vi "Read I2C.vi"(5 "Address":u8, 6 "NoStop (F)":bool, 7 "Bus":u8, 8 "error in (no error)":errorcluster, 9 "Len":u8, 11 "VISA resource name in":refnum<visa-resource-name>) -> (0 "error out":errorcluster, 1 "Data":string, 3 "VISA resource name":refnum<visa-resource-name>)   [LabVIEW 2024, in "CTIPicoVISA.lvlib"]
uses:
  CTIPicoVISA.lvlib
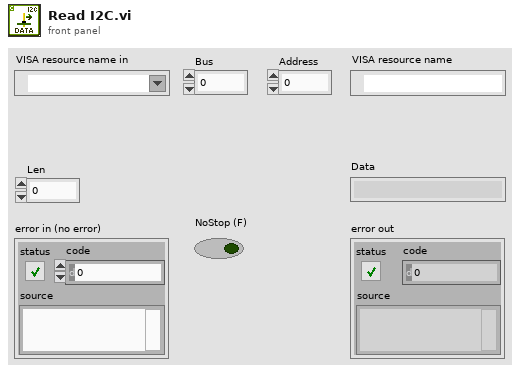
[diagram p1: front panel]
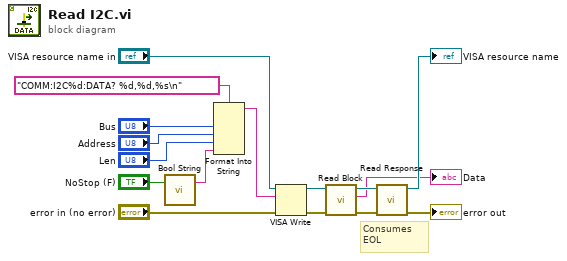
[diagram p0: block diagram]
diagram:
  # "Consumes EOL"
  n1 = call "Bool String.vi"("Bool"="NoStop (F)") -> ("String"=w3:string)  [unwired: 6 in]
  n2 = Format Into String(format string="COMM:I2C%d:DATA? %d,%d,%s\n", "Bus", "Address", "Len", w3) -> (resulting string=w1:string)  [unwired: 2 in, 1 out]
  n3 = VISA Write(VISA resource name="VISA resource name in", write buffer=w1, error in (no error)="error in (no error)") -> (VISA resource name out=w10:refnum<visa-resource-name>, error out=w11:errorcluster)  [unwired: 1 out]
  n4 = call "Read Block.vi"("error in (no error)"=w11, "VISA resource name in"=w10) -> ("error out"=w9:errorcluster, "Data"=→"Data":string, "VISA resource name"=w8:refnum<visa-resource-name>)  [unwired: 7 in]
  n5 = call "Read Response.vi"("error in (no error)"=w9, "VISA resource name"=w8) -> ("error out"=→"error out":errorcluster, "VISA resource name Out"=→"VISA resource name":refnum<visa-resource-name>)  [unwired: 6 in, 2 out]
